vi "Start_Switch_OFF.vi"(2 "Fail":bool, 3 "Pass":bool, 8 "error in (no error)":errorcluster) -> (0 "error out":errorcluster)   [LabVIEW 2020]
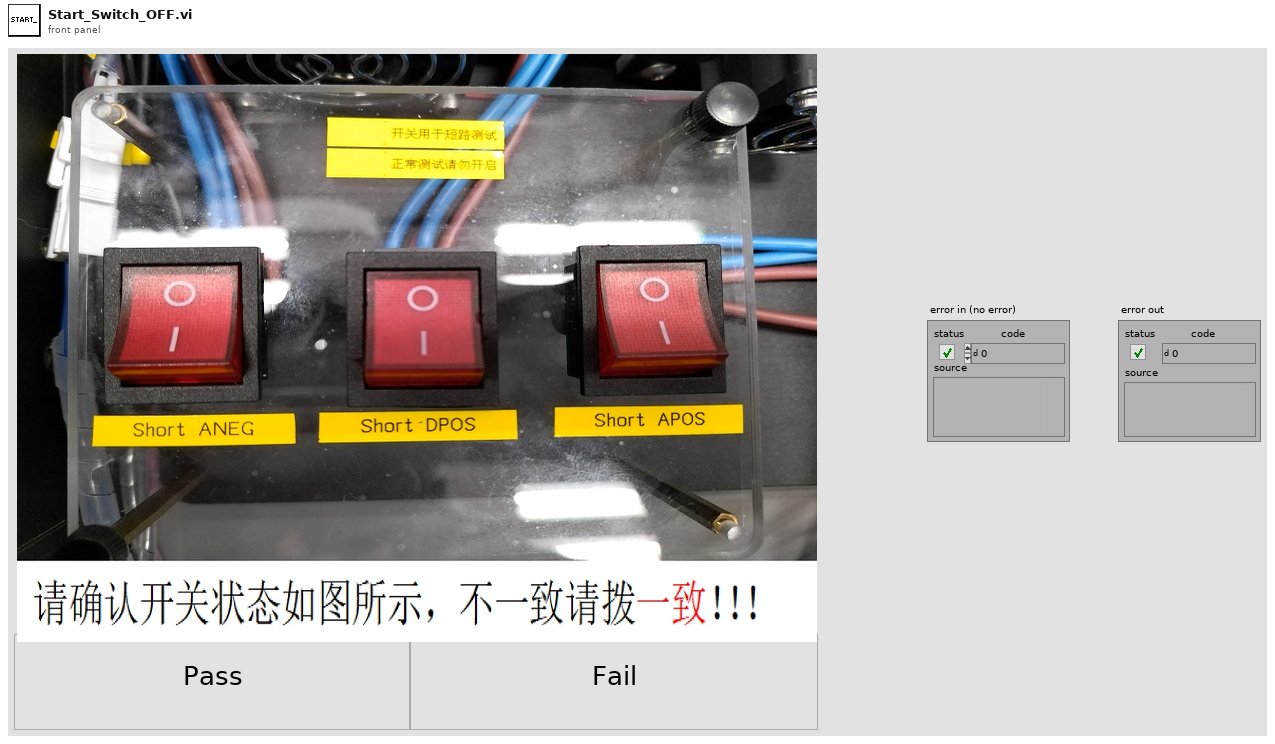
[diagram p1: front panel]
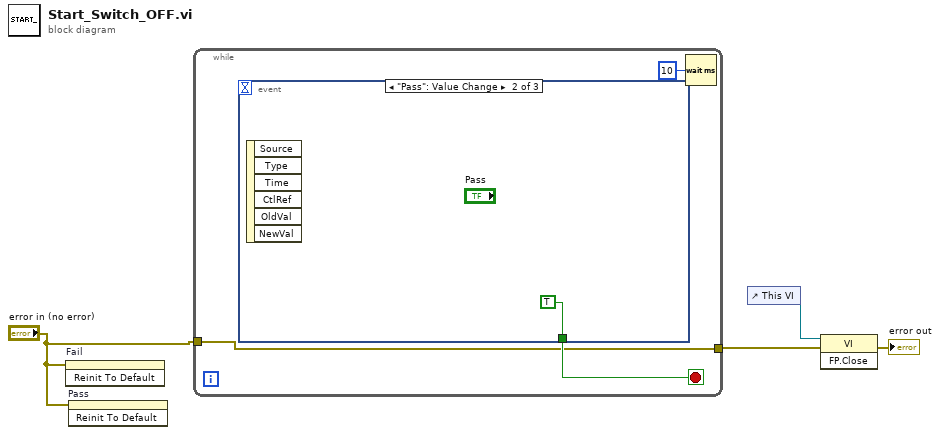
[diagram p0: block diagram]
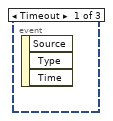
[diagram p2: hidden frame]
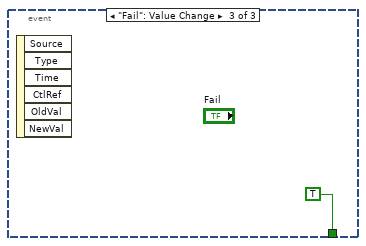
[diagram p3: hidden frame]
diagram:
  n1 = invoke on="Fail" class="Bool" method="Reinit To Default"(error in="error in (no error)") -> ()  [unwired: 2 in, 3 out]
  n2 = invoke on="Pass" class="Bool" method="Reinit To Default"(error in="error in (no error)") -> ()  [unwired: 2 in, 3 out]
  n3 = while {
    tunnel: "error in (no error)" -> [w5]
    tunnel: [w5] -> w2
    stop <- w7 stop-if-true
    n4 = event shown="[1] \"Pass\": Value Change" {
      selector: _ -> [_ _ _]
      dyn-events: _ -> [_ _ _]
      timeout: _ -> [_ _ _]
      tunnel: [_ TRUE TRUE] -> w7
      event Timeout {
        n5 = event-data() -> ()  [unwired: 1 in, 3 out]
      }
      event "Pass": Value Change {
        n6 = event-data() -> ()  [unwired: 1 in, 6 out]
      }
      event "Fail": Value Change {
        n7 = event-data() -> ()  [unwired: 1 in, 6 out]
      }
    }
    n8 = Wait (ms)(milliseconds to wait=u32 10) -> ()  [unwired: 1 out]
  }
  n9 = control-ref of="This VI"() -> (w3:refnum<vi>)
  n10 = invoke class="VI" method="FP.Close"(reference=w3, error in=w2) -> (error out=→"error out":errorcluster)  [unwired: 1 in, 2 out]
